vi "NI VeriStand - Get Waveform Data Reference.vi"(8 "error in (no error)":errorcluster, 11 "Waveform Ref in":T2=18446744073709551615 format="%.0x") -> (0 "error out":errorcluster, 2 "Waveform Data Reference":T1, 3 "Waveform Ref out":T2=18446744073709551615 format="%.0x")   [LabVIEW 2020, in "Custom Device API.lvlib"]
doc: "Returns a data reference for a specific waveform item in a custom device. Use waveform data references to open a session that reads from or writes to the waveform."
uses:
  <vilib>/NI VeriStand/Custom Device API/Custom Device API.lvlib
  <vilib>/NI VeriStand/Custom Device API/Custom Device Item Ref.ctl
  <vilib>/NI VeriStand/Custom Device API/Waveform Data Reference.ctl
  56b4e606-840f-4522-a59e-92a2d281d2b2.vi
  <vilib>/NI VeriStand/Custom Device API/Custom Device Offline Path.vi
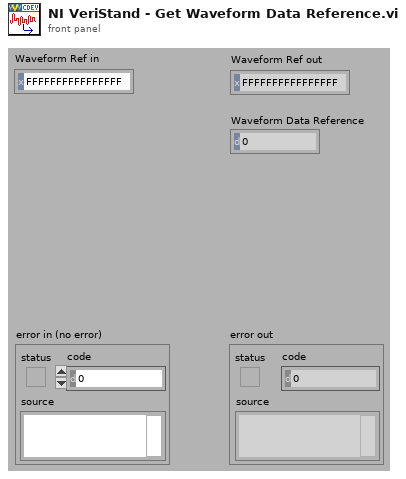
[diagram p1: front panel]
types:
  T1 = typedef "Custom Device API.lvlib/Waveform Data Reference.ctl" = i32
  T2 = typedef "Custom Device API.lvlib/Custom Device Item Ref.ctl" = u64
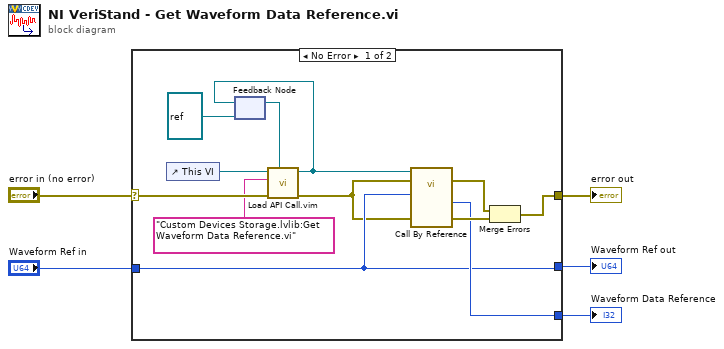
[diagram p0: block diagram]
diagram:
  n1 = case shown="No Error" "error in (no error)" {
    selector: "error in (no error)" -> [w10 w19]
    tunnel: [w16 w19] -> w5
    tunnel: "Waveform Ref in" -> [w14 w18]
    tunnel: [w14 w18] -> w3
    tunnel: [w15 _] -> w2
    frame No Error {
      n2 = control-ref of="This VI"() -> (w12:refnum<vi>)
      n3 = feedback #1(refnum<vi> refnum ("type specifier VI Refnum (for type only)")) -> (w13:refnum<vi>)
      n4 = call "Load API Call.vim"("VI reference in"=w13, "error in (no error)"=w10, "VI qualified name"="Custom Devices Storage.lvlib:Get Waveform Data Reference.vi", "Caller VI ref"=w12) -> ("error out"=w11:errorcluster, "VI reference"=w7:refnum<vi>)  [unwired: 6 in]
      n5 = feedback-in #1(w7) -> ()
      n6 = call-by-ref "?"(reference=w7, error in=w11, 8:"error in (no error)"=w11, "Waveform Ref in"=w14) -> (error out=w6:errorcluster, 0:"error out"=w17:errorcluster, "Waveform Data Reference"=w15:T1)  [unwired: 7 in, 2 out]
      n7 = Merge Errors(w6, w17) -> (w16:errorcluster)
    }
    frame Error {
    }
  }
  "error out" <- w5
  "Waveform Ref out" <- w3
  "Waveform Data Reference" <- w2
